vi "Set DO Pin.vi"(0 "RedPitaya connection in":refnum<k5>, 2 "Pin name":string, 3 "State":bool, 5 "error in":errorcluster, 12 "timeout ms (2000)":i32=2000) -> (14 "RedPitaya connection out":refnum<k5>, 19 "error out":errorcluster)   [LabVIEW 2010, in "RedPitaya.lvlib"]
doc: "Set state of digital outputs to True(HIGH) or False(LOW)."
uses:
  RedPitaya.lvlib
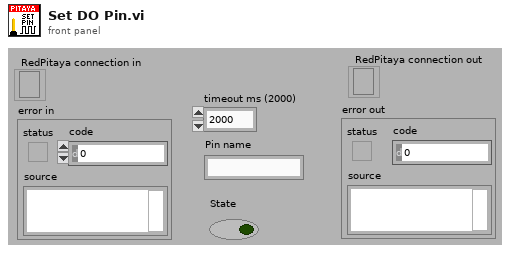
[diagram p1: front panel]
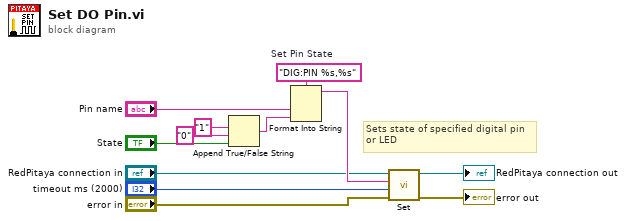
[diagram p0: block diagram]
diagram:
  w12 = "DIG:PIN %s,%s"  # Set Pin State
  # "Sets state of specified digital pin\nor LED"
  n1 = Append True/False String(1:"State", 2:"0" ("false string"), 3:"1" ("true string")) -> (0:w3:string)  [unwired: 1 in]
  n2 = Format Into String(format string=w12, "Pin name", w3) -> (resulting string=w11:string)  [unwired: 2 in, 1 out]
  n3 = call "Set.vi"("error in"="error in", "timeout ms (2000)"="timeout ms (2000)", "SCPI Message"=w11, "RedPitaya connection in"="RedPitaya connection in") -> ("error out"=→"error out":errorcluster, "RedPitaya connection out"=→"RedPitaya connection out":refnum<k5>)  [unwired: 5 in, 1 out]
